vi "GLIMPSE Get image from disk.vi"(5 "Header file data":T1 {"Pixel depth" items=["8 bits", "16 bits", "Float", "Complex", "RGB", "HSL"]; "time of 1st frame, \nsec since 1/1/04" format="%.2f"}, 6 "error in":errorcluster, 7 "Acqisition files refnums":refnum<file>[](array[refnum]), 9 "Physical Frame Number\n(Starting with zero)":u32, 10 "Image buffer in":T5) -> (0 "error out":errorcluster, 3 "Image out":T5)   [LabVIEW 2016]
doc: "Extracts a single frame from the acquired image disk store."
uses:
  <vilib>/vision/Image Controls.llb/IMAQ Image.ctl
  Header file data.ctl
  Seq file v 1/Offset table.ctl
  Seq file v 1/Offset.ctl
  Seq file v 1/file number.ctl
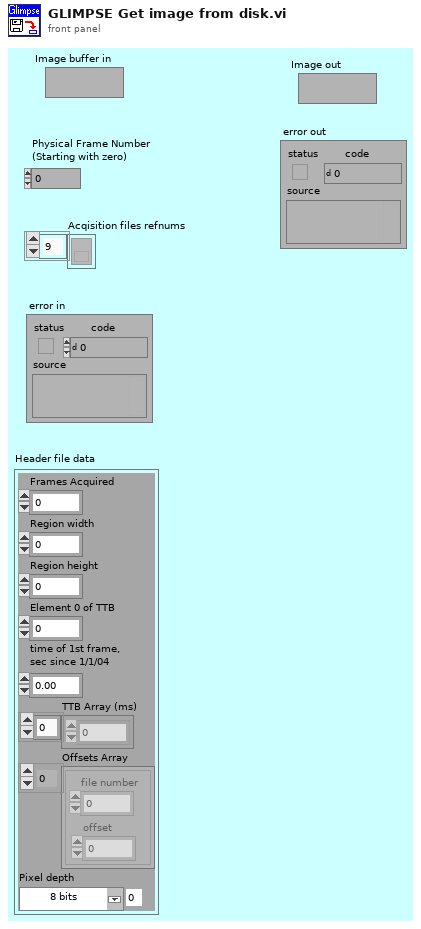
[diagram p1: front panel]
types:
  T1 = typedef "Header file data.ctl" = cluster{"Frames Acquired":u32, "Region width":i32, "Region height":i32, "Element 0 of TTB":u32, "time of 1st frame, \nsec since 1/1/04":dbl, "TTB Array (ms)":u32[], "Offsets Array":T2, "Pixel depth":u32}
  T2 = typedef "Offset table.ctl" = cluster{"offset":T3, "file number":T4}[]
  T3 = typedef "Offset.ctl" = i32
  T4 = typedef "file number.ctl" = u8
  T5 = typedef "IMAQ Image.ctl" = refnum<image>
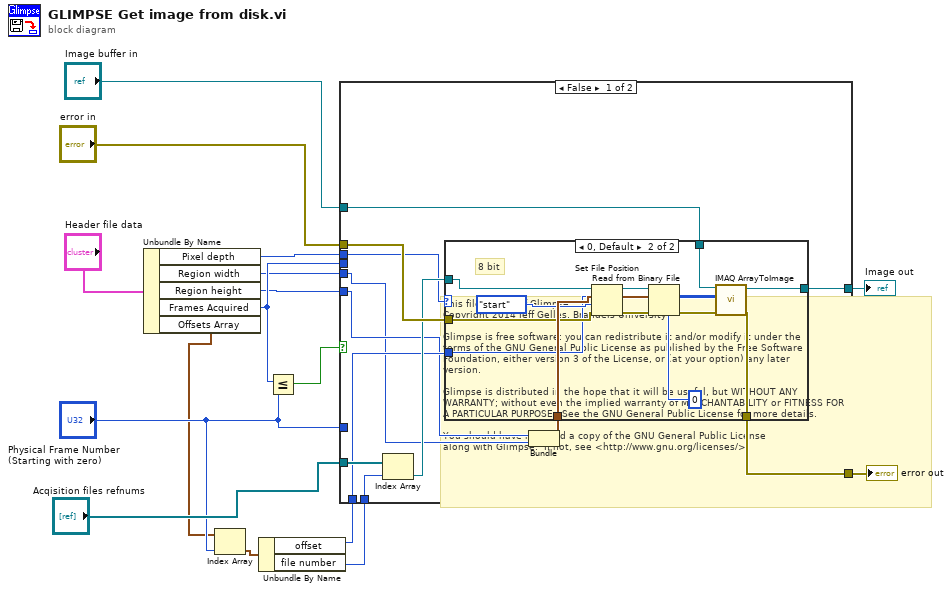
[diagram p0: block diagram]
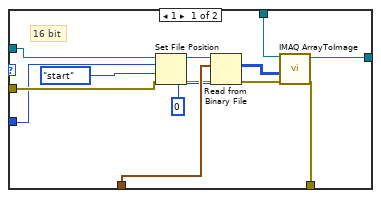
[diagram p2: hidden frame]
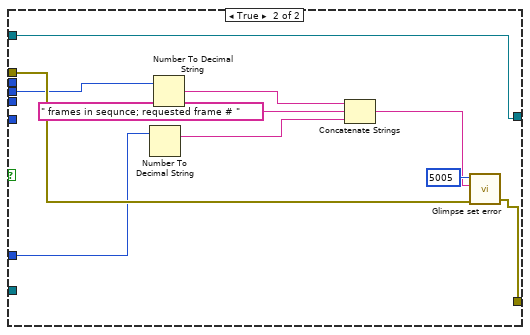
[diagram p3: hidden frame]
diagram:
  # "This file is part of Glimpse. \nCopyright 2014 Jeff Gelles, Brandeis University.    \n\nGlimpse is free software: you can redistribute it and/or modify it under the \nterms of the GNU General Public License as published by the Free Software \nFoundation, either version 3 of the License, or (at your option) any later \nversion.\n\nGlimpse is distributed in the hope that it will be useful, but WITHOUT ANY \nWARRANTY; without even the implied warranty of MERCHANTABILITY or FITNESS FOR \nA PARTICULAR PURPOSE.  See the GNU General Public License for more details.\n\nYou should have received a copy of the GNU General Public License\nalong with Glimpse.  If not, see <http://www.gnu.org/licenses/>."
  n1 = Unbundle By Name("Header file data") -> ("Pixel depth"=w5:u32, "Region width"=w1:i32, "Region height"=w2:i32, "Frames Acquired"=w4:u32, "Offsets Array"=w3:T2)
  n2 = Index Array(array=w3, index="Physical Frame Number\n(Starting with zero)") -> (element=w10:cluster{"offset":T3, "file number":T4})
  n3 = Unbundle By Name(w10) -> ("offset"=w8:T3, "file number"=w9:T4)
  n4 = Less Or Equal?(x=w4, y="Physical Frame Number\n(Starting with zero)") -> (x <= y?=w11:bool)
  n5 = case shown="False" w11 {
    tunnel: "Image buffer in" -> [w27 w64]
    tunnel: "error in" -> [w26 w62]
    tunnel: [w24 w64] -> w14
    tunnel: [w25 w63] -> w13
    tunnel: "Acqisition files refnums" -> [w23 _]
    tunnel: w9 -> [w21 _]
    tunnel: w8 -> [w20 _]
    tunnel: w4 -> [_ w57]
    tunnel: "Physical Frame Number\n(Starting with zero)" -> [_ w55]
    tunnel: w5 -> [w19 _]
    tunnel: w2 -> [w18 _]
    tunnel: w1 -> [w17 _]
    frame False {
      n6 = Index Array(array=w23, index=w21) -> (element=w22:refnum<file>)
      n7 = Bundle("Region height"=w18, "Region width"=w17) -> (w28:cluster{"Region height":i32, "Region width":i32})  [unwired: 1 out]
      n8 = case shown="0, Default" w19 {
        tunnel: w28 -> [w41 w53]
        tunnel: w27 -> [w38 w50]
        tunnel: w26 -> [w37 w49]
        tunnel: [w36 w48] -> w25
        tunnel: [w35 w47] -> w24
        tunnel: w22 -> [w29 w46]
        tunnel: w20 -> [w34 w45]
        frame 1 {
          # "16 bit"
          n9 = Set File Position(offset (in bytes) (0)=w34, refnum=w29, from (0:start)=enum16{"start", "end", "current"}."start" ("pos mode (0:2)"), error in=w37) -> (refnum out=w31:refnum<file>, error out=w30:errorcluster)
          n10 = Read from Binary File(5:i16 0 ("byte stream type"), 8:w30, 10:w41, 11:w31) -> (0:w33:errorcluster, 2:w32:i16[][])  [unwired: 4 out]
          n11 = call "IMAQ ArrayToImage"("error in (no error)"=w33, "Image Pixels (I16)"=w32, "Image"=w38) -> ("error out"=w36:errorcluster, "Image Out"=w35:T5)  [unwired: 3 in, 4 out]
        }
        frame 0, Default {
          # "8 bit"
          n12 = Set File Position(offset (in bytes) (0)=w45, refnum=w46, from (0:start)=enum16{"start", "end", "current"}."start" ("pos mode (0:2)"), error in=w49) -> (refnum out=w43:refnum<file>, error out=w42:errorcluster)
          n13 = Read from Binary File(5:u8 0 ("byte stream type"), 8:w42, 10:w53, 11:w43) -> (0:w44:errorcluster, 2:w54:u8[][])  [unwired: 4 out]
          n14 = call "IMAQ ArrayToImage"("error in (no error)"=w44, "Image Pixels (U8)"=w54, "Image"=w50) -> ("error out"=w48:errorcluster, "Image Out"=w47:T5)  [unwired: 3 in, 4 out]
        }
      }
    }
    frame True {
      n15 = Number To Decimal String(number=w55) -> (decimal integer string=w56:string)  [unwired: 1 out]
      n16 = Number To Decimal String(number=w57) -> (decimal integer string=w58:string)  [unwired: 1 out]
      n17 = Concatenate Strings(w58, " frames in sequnce; requested frame # " ("string"), w56) -> (w60:string)
      n18 = call "Glimpse set error.vi"("code"=5005, "Additional information"=w60, "error in"=w62) -> ("error out"=w63:errorcluster)  [unwired: 5 out]
    }
  }
  "Image out" <- w14
  "error out" <- w13
